vi "计时.vi"(9 "单位":dbl, 10 "初始化":bool, 11 "计时时间(s)":dbl) -> (2 "完成 2":dbl, 3 "完成":bool)   [LabVIEW 2017]
panel:
  out "数值":i32
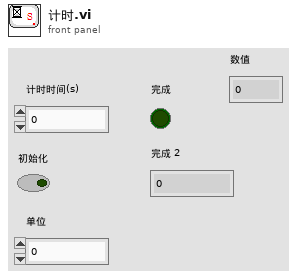
[diagram p1: front panel]
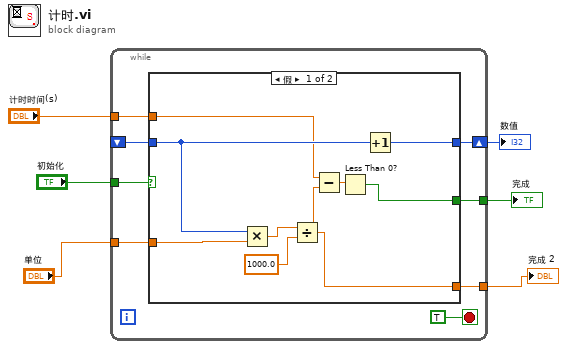
[diagram p0: block diagram]
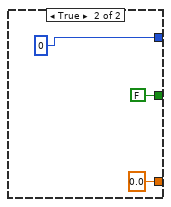
[diagram p2: hidden frame]
diagram:
  n1 = while {
    tunnel: "初始化" -> [w13]
    shift-right: [w12] -> w1
    shift-left: _ -> [w11]
    tunnel: "计时时间(s)" -> [w10]
    tunnel: "单位" -> [w9]
    tunnel: [w8] -> w3
    tunnel: [w7] -> w2
    stop <- TRUE stop-if-true
    n2 = case shown="假" w13 {
      tunnel: [w15 0] -> w12
      tunnel: w11 -> [w20 _]
      tunnel: w10 -> [w19 _]
      tunnel: w9 -> [w18 _]
      tunnel: [w17 FALSE] -> w8
      tunnel: [w16 0.0] -> w7
      frame False {
        n3 = Multiply(x=w20, y=w18) -> (x*y=w23:dbl)
        n4 = Divide(x=w23, y=1000.0 ("x")) -> (x/y=w16:dbl)
        n5 = Subtract(x=w19, y=w16) -> (x-y=w21:dbl)
        n6 = Less Than 0?(x=w21) -> (x < 0?=w17:bool)
        n7 = Increment(x=w20) -> (x+1=w15:i32)
      }
      frame True {
      }
    }
  }
  "完成" <- w3
  "完成 2" <- w2
  "数值" <- w1
